vi "Get Column String.vi"(8 "error in (no error)":errorcluster, 11 "PQ Result  in":refnum<class "PQ Result.lvclass">) -> (0 "error out":errorcluster, 2 "String":string, 3 "PQ Result  out":refnum<class "PQ Result.lvclass">)   [LabVIEW 2015, in "PQ Result.lvclass"]
uses:
  PQ Result.lvclass
  PQ Result.lvclass/PQ Result.ctl
  <vilib>/LAVA/_libpq_internal_deps/libpq.dll
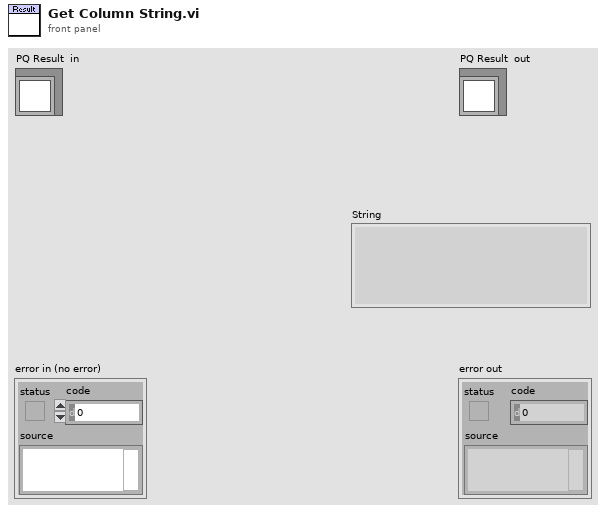
[diagram p1: front panel]
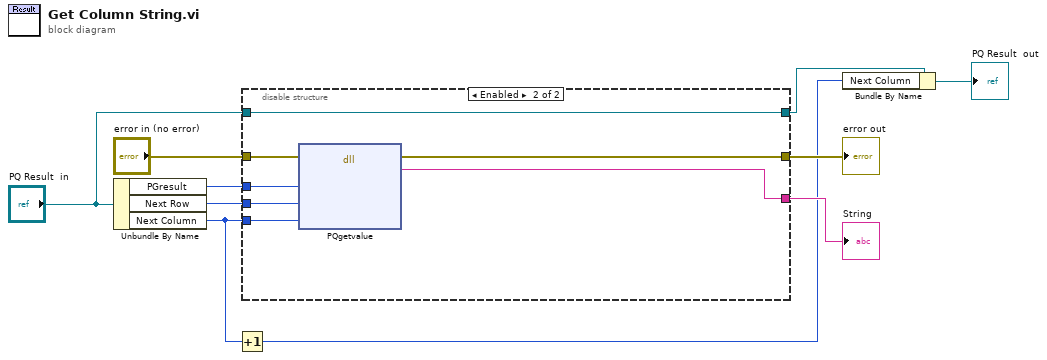
[diagram p0: block diagram]
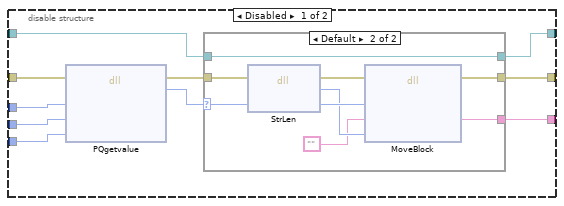
[diagram p2: hidden frame]
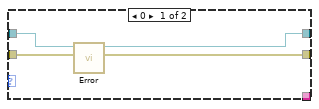
[diagram p3: hidden frame]
diagram:
  n1 = Unbundle By Name("PQ Result  in") -> ("PGresult"=w8:u32, "Next Row"=w6:i32, "Next Column"=w4:i32)
  n2 = Increment(x=w4) -> (x+1=w3:i32)
  n3 = disable-structure shown="Enabled" {
    disable-tunnel: "error in (no error)" -> [w20 w40]
    disable-tunnel: [w19 w36] -> w9
    disable-tunnel: w8 -> [w18 w39]
    disable-tunnel: [w15 w34] -> w7
    disable-tunnel: w6 -> [w14 w38]
    disable-tunnel: w4 -> [w13 w37]
    disable-tunnel: "PQ Result  in" -> [w12 w35]
    disable-tunnel: [w11 w35] -> w1
    frame Disabled {
      n4 = dll-call lib="C:/Program Files (x86)/National Instruments/LabVIEW 2015/vi.lib/LAVA/_libpq_internal_deps/libpq.dll" fn="PQgetvalue"(error in=w20, "PGresult"=w18, "row_number"=w14, "column_number"=w13) -> (error out=w16:errorcluster, "PQgetvalue_ptr"=w17:u32)  [unwired: 5 in, 1 out]
      n5 = case shown="Default" w17 {
        selector: w17 -> [_ w26]
        tunnel: w16 -> [w24 w33]
        tunnel: [w23 w31] -> w19
        tunnel: [_ w28] -> w15
        tunnel: w12 -> [w22 w25]
        tunnel: [w21 w25] -> w11
        frame 0 {
          n6 = call "Error.vi"("error in (no error)"=w24, "PQ Result  In"=w22) -> ("error out"=w23:errorcluster, "PQ Result"=w21:refnum<class "PQ Result.lvclass">)  [unwired: 8 in]
        }
        frame Default {
          n7 = dll-call lib="LabVIEW" fn="StrLen"(error in=w33, "p_src"=w26) -> (error out=w32:errorcluster, "str_len"=w29:u32, "p_src"=w30:u32)  [unwired: 2 in, 1 out]
          n8 = dll-call lib="LabVIEW" fn="MoveBlock"(error in=w32, "p_src"=w30, "dst"="", "size"=w29) -> (error out=w31:errorcluster, "dst"=w28:string)  [unwired: 5 in, 1 out]
        }
      }
    }
    frame Enabled {
      n9 = dll-call lib="C:/Program Files (x86)/National Instruments/LabVIEW 2015/vi.lib/LAVA/_libpq_internal_deps/libpq.dll" fn="PQgetvalue"(error in=w40, "PGresult"=w39, "row_number"=w38, "column_number"=w37) -> (error out=w36:errorcluster, "PQgetvalue"=w34:string)  [unwired: 5 in, 1 out]
    }
  }
  "error out" <- w9
  "String" <- w7
  n10 = Bundle By Name(cluster=w1, "Next Column"=w3) -> (→"PQ Result  out":refnum<class "PQ Result.lvclass">)
